vi "SetRange.vi"(8 "Sleep":u32=200, 9 "DoIt":bool=TRUE, 10 "Range":T1) -> (0 "Sleep":u32)   [LabVIEW 2025]
uses:
  Range.ctl
  Globals.vi
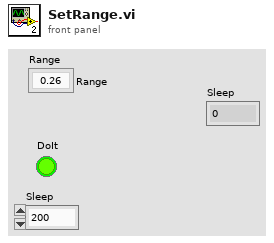
[diagram p1: front panel]
types:
  T1 = typedef "Range.ctl" = enum16{"0.26", "0.52", "1.03", "2.05", "4.1", "6.2"}
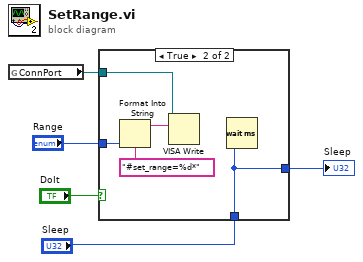
[diagram p0: block diagram]
diagram:
  n1 = global read "Globals.vi" "ConnPort"() -> (w1:refnum<visa-resource-name>)
  n2 = case shown="True" "DoIt" {
    tunnel: [w6 w7] -> w5
    tunnel: "Range" -> [_ w11]
    tunnel: w1 -> [_ w10]
    tunnel: "Sleep" -> [w6 w7]
    frame False {
    }
    frame True {
      n3 = Format Into String(format string="#set_range=%d*", w11) -> (resulting string=w9:string)  [unwired: 2 in, 1 out]
      n4 = VISA Write(VISA resource name=w10, write buffer=w9) -> ()  [unwired: 1 in, 3 out]
      n5 = Wait (ms)(milliseconds to wait=w7) -> ()  [unwired: 1 out]
    }
  }
  "Sleep" <- w5
